vi "MCL Setup Read Wave Form N.vi"(7 "handle":i32, 9 "milliseconds":dbl, 10 "DataPoints":u32, 11 "axis":u32) -> (3 "function return":i32)   [LabVIEW 2017, in "Madlib.lvlib"]
doc: "MADLIB_API int MCL_Setup_ReadWaveFormN(unsigned int axis,unsigned int DataPoints,double milliseconds, int handle);"
uses:
  Madlib.lvlib
  Madlib.dll
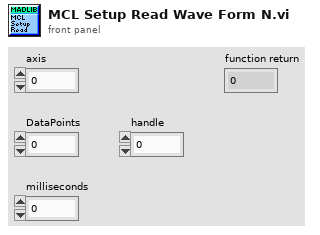
[diagram p1: front panel]
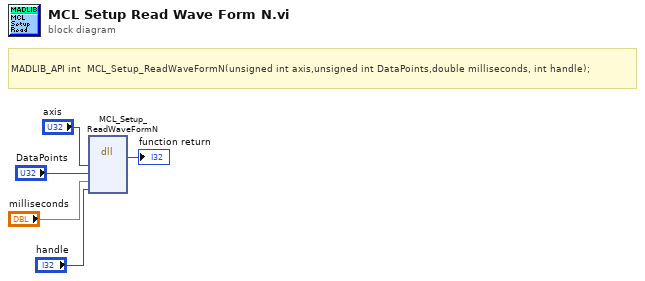
[diagram p0: block diagram]
diagram:
  # "MADLIB_API\tint\t\tMCL_Setup_ReadWaveFormN(unsigned int axis,unsigned int DataPoints,double milliseconds, int handle);"
  n1 = dll-call lib="C:/Users/francesco/dev/pump-probe/Piezo/lvlib/Madlib.*" fn="MCL_Setup_ReadWaveFormN"("axis"="axis", "DataPoints"="DataPoints", "milliseconds"="milliseconds", "handle"="handle") -> (→"function return":i32)  [unwired: 7 in, 2 out]
